vi "pulse_tester.vi"() -> ()   [LabVIEW 2021]
uses:
  CTL/emitter params.ctl
  CTL/mode_type.ctl
  pdw.ctl
  <vilib>/measure/maspectr.llb/FFT Power Spectrum and PSD for 1 Chan (CDB).vi
  <vilib>/Analysis/NI_AALPro.lvlib
  <vilib>/measure/NI_MAPro.lvlib
  <instrlib>/_niInstr/Basic Elements/v1/FPGA/niInstr Basic Elements v1 FPGA.lvlib
panel:
  out "D phase to Dt":dbl[](graph)
  out "output valid":i16[](graph)
  in  "tx rate":i32=50
  out "Cluster":T1={"PW"=60000, "frequency shift"=0.004999999999999005, "amp"=0.31623077392578125, "mode type"=enum."LFM", "mode depth"=234562481, "mode filter"=0, "phase shift"=0.0, "pulse shape filter"=0}
  out "Array":i32[](array[numeric])
  out "free DDS":i16[](graph)
  out "Power Spectrum / PSD":cluster{"f0":dbl, "df":dbl, "magnitude":dbl[]}[](graph)
  out "amp out":dbl[](graph)
  out "phase out":dbl[](graph)
  in  "num of sampels for test":i32=30000 format="%.0p"
  out "I data":dbl[](graph)
  in  "emmiter":T3[](array[typedef])=[{"f set"=[1000000.0], "hop rate (Hz)"=1000.0, "d.c."=0.001, "amp (dB)"=-10.0, "mod type"=enum."CW", "mod depth"=10000000.0, "DOA"=0.0, "t start"=0.0, "t end"=3.0}] {"t end" format="%#_3p"; "t start" format="%#_3p"; "DOA" format="%#_3p"; "mod depth" format="%.0p"}
  out "phase in to DDS":dbl[](graph)
  out "frequncy  in to DDS":dbl[](graph)
  in  "Fs":i32=200000000 format="%.0p"
  # "mode type:\n0- cw\n3-lfm\n4- bpsk\n5-qpsk"
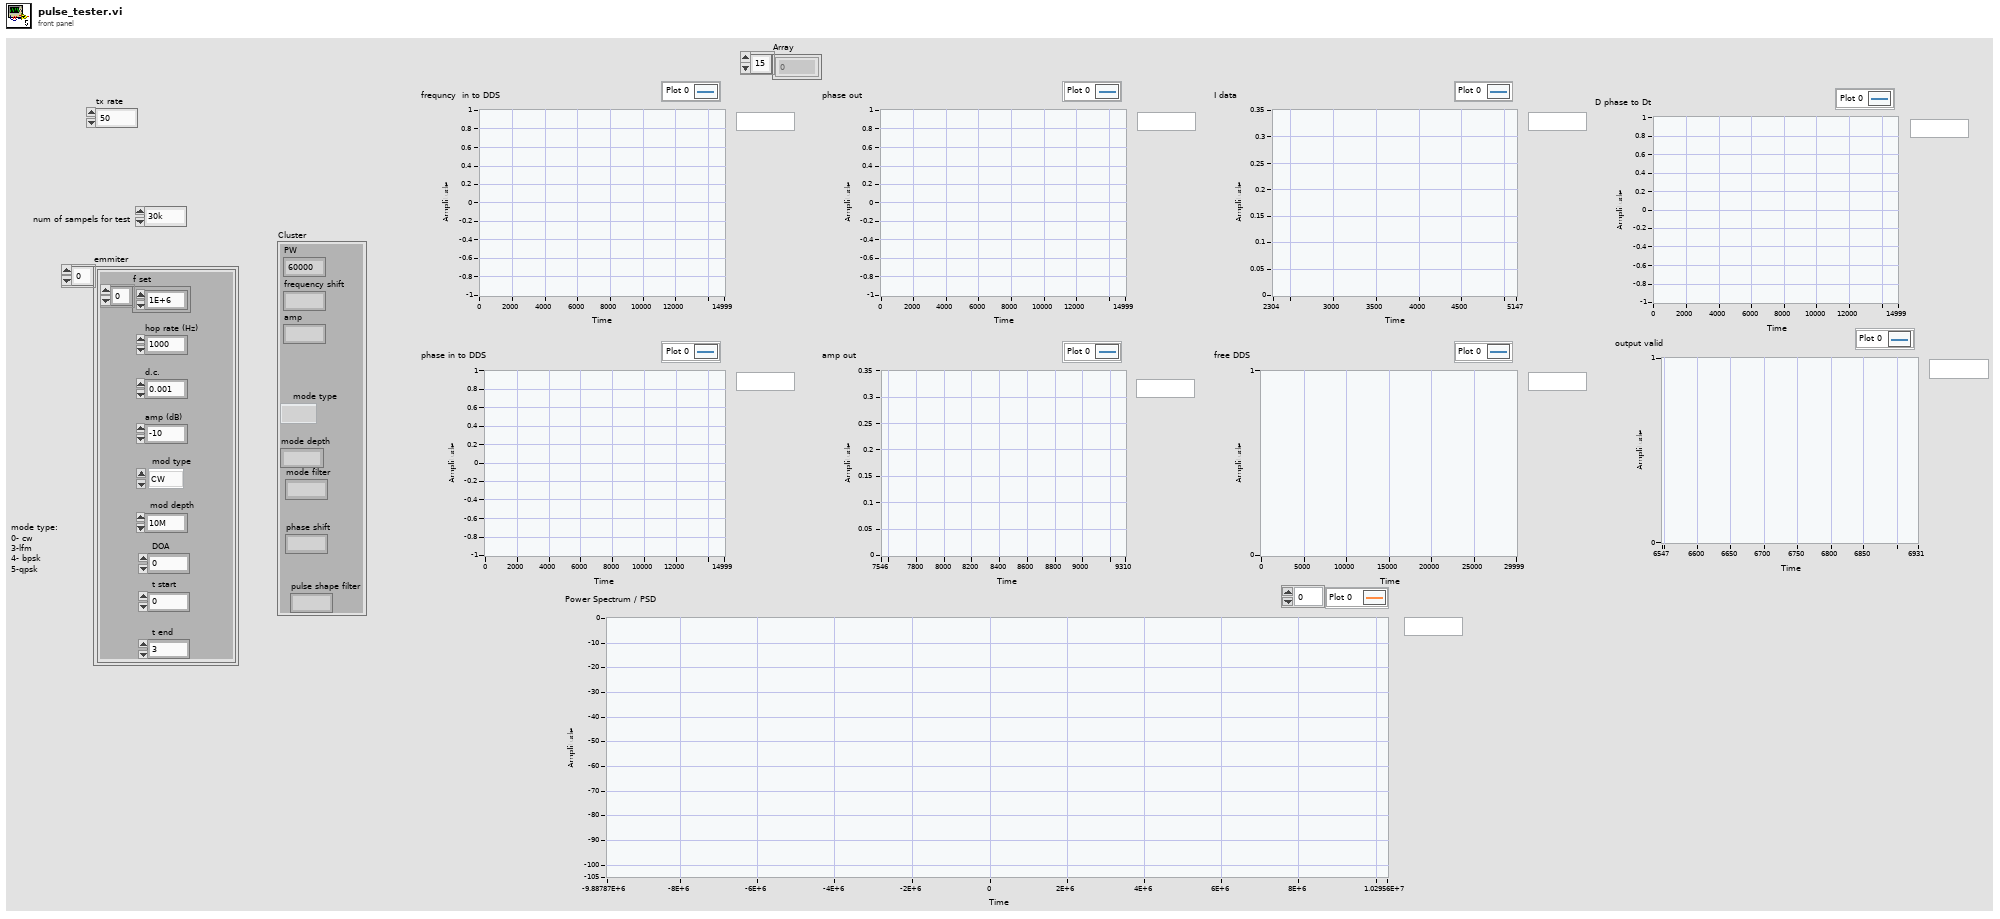
[diagram p1: front panel]
types:
  T1 = typedef "pdw.ctl" = cluster{"PW":u32, "frequency shift":fxp<+/-,48,0>, "amp":fxp<+/-,18,1>, "mode type":T2, "mode depth":u32, "mode filter":u8, "phase shift":fxp<+/-,16,1>, "pulse shape filter":u8}
  T2 = typedef "mode_type.ctl" = enum8{"CW", "from memory 1", "NC - cw", "LFM", "BPSK", "QPSK"}
  T3 = typedef "emitter params.ctl" = cluster{"f set":dbl[], "hop rate (Hz)":dbl, "d.c.":dbl, "amp (dB)":dbl, "mod type":T2, "mod depth":dbl, "DOA":dbl, "t start":dbl, "t end":dbl}
  T4 = typedef "PDW_lv2.ctl" = cluster{"t start":dbl, "frequency (Hz)":dbl, "duration (sec)":dbl, "amp (lin)":dbl, "mod type":T2, "mod depth":dbl, "phase (rad)":dbl[]}
  T5 = typedef "niInstr DSP v1 Shared.lvlib/IQ Data.ctl" = cluster{"I":fxp<+/-,18,1>, "Q":fxp<+/-,18,1>, "overflow":bool}
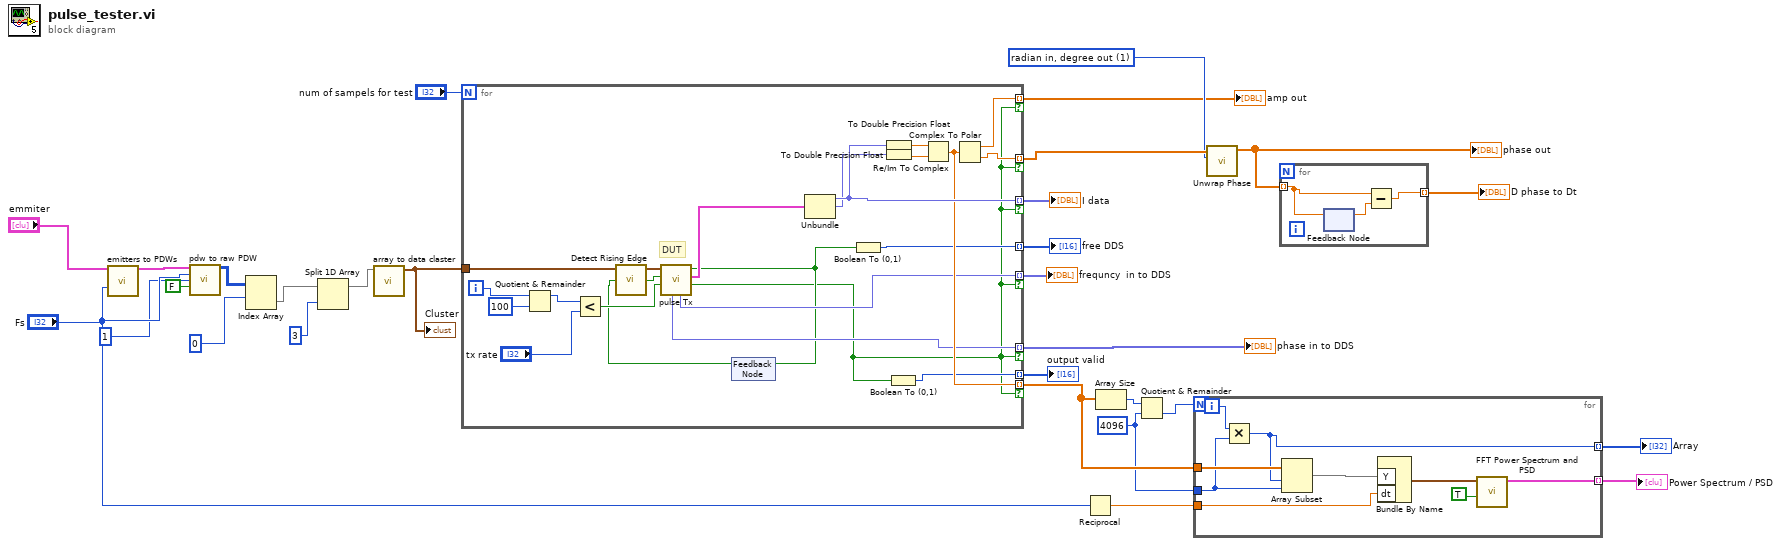
[diagram p0: block diagram]
diagram:
  w14 = 4096 ("length")
  w25 = 1 items=["radian in, radian out", "radian in, degree out", "degree in, degree out", "degree in, radian out"] ("phase unit")
  n1 = call "emitters to PDWs.vi"("emmiter"="emmiter", "center frequency (Hz)"="Fs") -> ("sorted array"=w22:T4[])  [unwired: 11 in, 2 out]
  n2 = call "pdw to raw PDW.vi"("PDWs"=w22, "Fs fpGa"="Fs", "SPC"=1, "gen for DF"=FALSE) -> ("Array"=w8:u64[][])  [unwired: 9 in, 2 out]
  n3 = Index Array(array=w8, index (row)=0) -> (element=w3:u64[])  [unwired: 1 in]
  n4 = Split 1D Array(array=w3, index=3) -> (first subarray=w1:u64[])  [unwired: 1 out]
  n5 = call "array to data claster.vi"("Array"=w1) -> ("Cluster"=w18:T1)  [unwired: 10 in]
  "Cluster" <- w18
  n6 = for {
    N: "num of sampels for test" -> [_]
    tunnel: [w50] -> w29 mode=indexing if=w30
    tunnel: [w40] -> w28 mode=indexing if=w30
    tunnel: [w41] -> w27 mode=indexing if=w30
    tunnel: [w46] -> w26 mode=indexing if=w30
    tunnel: [w47] -> w24 mode=indexing if=w30
    tunnel: w18 -> [w49]
    tunnel: [w45] -> w20 mode=indexing if=w30
    tunnel: [w44] -> w17 mode=indexing
    tunnel: [w33] -> w11 mode=indexing
    i -> [w38]
    # "DUT"
    n7 = Quotient & Remainder(x=w38, y=100) -> (x-y*floor(x/y)=w36:i32)  [unwired: 1 out]
    n8 = Less?(x=w36, y="tx rate") -> (x < y?=w34:bool)
    n9 = feedback #1() -> (w32:bool)  [unwired: 1 in]
    n10 = call <instrlib>:"Detect Rising Edge.vi"("signal"=w32) -> ("edge detected"=w31:bool)  [unwired: 14 in]
    n11 = call "pulse Tx.vi"("enable line"=w34, "take it!"=w31, "Cluster"=w49) -> ("output valid"=w30:bool, "data out"=w51:T5, "free dds"=w39:bool, "frequncy"=w40:fxp<+/-,48,0>, "phase"=w41:fxp<+/-,16,1>)  [unwired: 4 in]
    n12 = feedback-in #1(w39) -> ()
    n13 = Unbundle(w51) -> ("I"=w50:fxp<+/-,18,1>, "Q"=w48:fxp<+/-,18,1>)  [unwired: 1 out]
    n14 = Boolean To (0,1)(Boolean=w39) -> (0, 1=w44:i16)
    n15 = To Double Precision Float(number=w50) -> (double precision float=w43:dbl)
    n16 = To Double Precision Float(number=w48) -> (double precision float=w42:dbl)
    n17 = Boolean To (0,1)(Boolean=w30) -> (0, 1=w33:i16)
    n18 = Re/Im To Complex(1:w42, 2:w43) -> (0:w45:cdb)
    n19 = Complex To Polar(r * e^(i*theta)=w45) -> (r=w47:dbl, theta=w46:dbl)
  }
  "frequncy  in to DDS" <- w28
  "phase in to DDS" <- w27
  "I data" <- w29
  "amp out" <- w24
  "free DDS" <- w17
  "output valid" <- w11
  n20 = Reciprocal(x="Fs") -> (1/x=w21:dbl)
  n21 = Array Size(array=w20) -> (size(s)=w15:i32)
  n22 = Quotient & Remainder(x=w15, y=w14) -> (floor(x/y)=w13:i32)  [unwired: 1 out]
  n23 = for {
    N: w13 -> [_]
    tunnel: w20 -> [w57]
    tunnel: w21 -> [w56]
    tunnel: w14 -> [w55]
    tunnel: [w53] -> w12 mode=indexing
    tunnel: [w54] -> w16 mode=indexing
    i -> [w52]
    n24 = Multiply(x=w52, y=w55) -> (x*y=w54:i32)
    n25 = Array Subset(array=w57, index=w54, length=w55) -> (w58:cdb[])
    n26 = Bundle By Name("Y"=w58, "dt"=w56) -> (w60:waveform(cdb))  [unwired: 1 in]
    n27 = call-poly <vilib>:"FFT Power Spectrum and PSD.vi"("dB On (F)"=TRUE, "time signal"=w60) -> ("Power Spectrum / PSD"=w53:cluster{"f0":dbl, "df":dbl, "magnitude":dbl[]})  [unwired: 6 in, 3 out]
  }
  "Power Spectrum / PSD" <- w12
  "Array" <- w16
  n28 = call <vilib>:"Unwrap Phase.vi"("phase unit"=w25, "Phase"=w26) -> ("Unwrapped Phase"=w10:dbl[])  [unwired: 8 in, 1 out]
  "phase out" <- w10
  n29 = for {
    tunnel: w10 -> [w63] mode=indexing
    tunnel: [w61] -> w9 mode=indexing
    n30 = feedback-in #2(w63) -> ()
    n31 = feedback #2() -> (w62:dbl)  [unwired: 1 in]
    n32 = Subtract(x=w63, y=w62) -> (x-y=w61:dbl)
  }
  "D phase to Dt" <- w9
